vi "Wildcard CONSTANT.vi"() -> (0 "input 1":string)   [LabVIEW 2009, in "Database Lib.lvlib"]
uses:
  Database Lib.lvlib
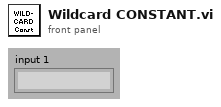
[diagram p1: front panel]
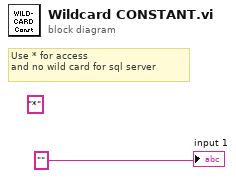
[diagram p0: block diagram]
diagram:
  (unwired) "*" ("input 1")
  # "Use * for access\nand no wild card for sql server"
  "input 1" <- "" ("input 1")
